vi "byv.vi"() -> ()   [LabVIEW 2011]
panel:
  out "z":dbl
  in  "y":dbl
  in  "x":dbl
  out "z":dbl
  in  "y":dbl
  in  "x":dbl
  out "z":dbl
  out "y":dbl
  in  "d":dbl
  in  "c":dbl
  in  "b":dbl
  in  "a":dbl
  out "differen":bool
  out "borrow":bool
  in  "c":bool
  in  "b":bool
  in  "a":bool
  in  "Boolean":bool
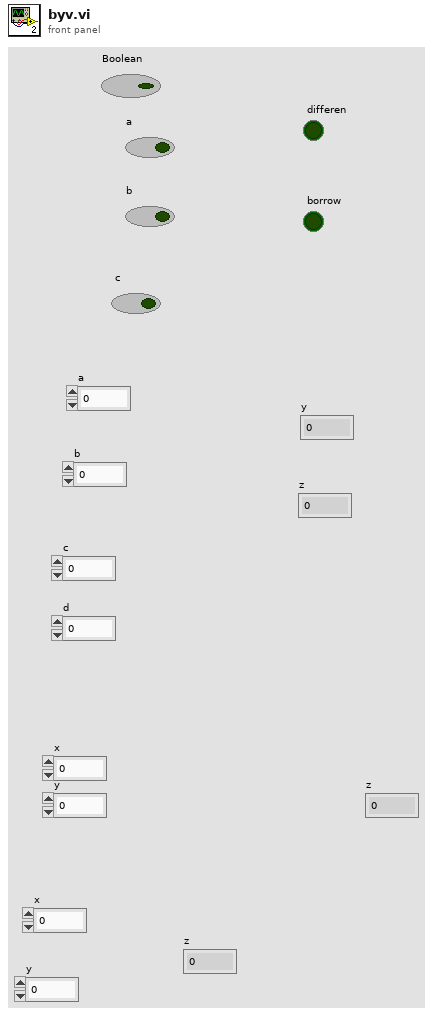
[diagram p1: front panel]
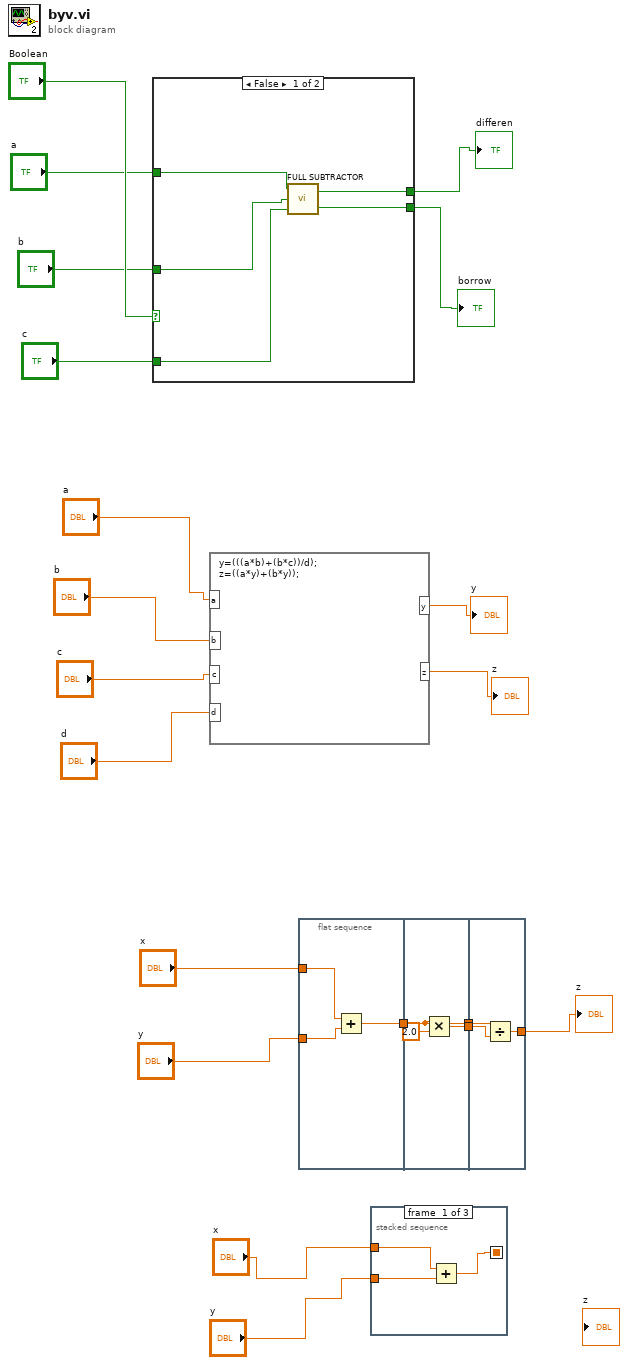
[diagram p0: block diagram]
diagram:
  n1 = case shown="False" "Boolean" {
    tunnel: "a" -> [w25 _]
    tunnel: "b" -> [w24 _]
    tunnel: "c" -> [w23 _]
    tunnel: [w22 _] -> w16
    tunnel: [w21 _] -> w15
    frame False {
      n2 = call "FULL SUBTRACTOR.vi"("C"=w23, "B"=w24, "A"=w25) -> ("BORROW"=w21:bool, "DIFF"=w22:bool)
    }
    frame True {
    }
  }
  "borrow" <- w15
  "differen" <- w16
  n3 = formula code="y=(((a*b)+(b*c))/d);\nz=((a*y)+(b*y));"("a"="a", "b"="b", "c"="c", "d"="d") -> ("y"=→"y":dbl, "z"=→"z":dbl)
  n4 = flat-sequence {
    tunnel: "x" -> [w28]
    tunnel: "y" -> [w27]
    tunnel: [w26] -> w6
    tunnel: w6 -> [w30]
    tunnel: [w30] -> w5
    tunnel: [w29] -> w4
    tunnel: w5 -> [w34]
    tunnel: w4 -> [w33]
    tunnel: [w32] -> w3
    frame #0 {
      n5 = Add(x=w28, y=w27) -> (x+y=w26:dbl)
    }
    frame #1 {
      n6 = Multiply(x=w30, y=2.0) -> (x*y=w29:dbl)
    }
    frame #2 {
      n7 = Divide(x=w34, y=w33) -> (x/y=w32:dbl)
    }
  }
  n8 = stacked-sequence {
    seq-local: [w35 _ _] -> [_ _ _]
    tunnel: "x" -> [w37 _ _]
    tunnel: "y" -> [w36 _ _]
    frame #0 {
      n9 = Add(x=w37, y=w36) -> (x+y=w35:dbl)
    }
    frame #1 {
    }
    frame #2 {
    }
  }
  "z" <- w3
